vi "test2.vi"() -> ()   [LabVIEW 2019]
uses:
  <vilib>/measure/NI_MABase.lvlib
panel:
  out "Button 2":dbl
  out "Button 1":dbl
  out "Y":dbl
  out "X":dbl
  in  "Frequeny":dbl(slide) scale=0.0..10.0
  in  "Amplitude":dbl(slide) scale=0.0..10.0
  in  "Power":bool
  out "Signal":dynamicdata(graph)
  in  "Sine":bool
  # "Remote gesture control enabled Control Panel"
  # "Square"
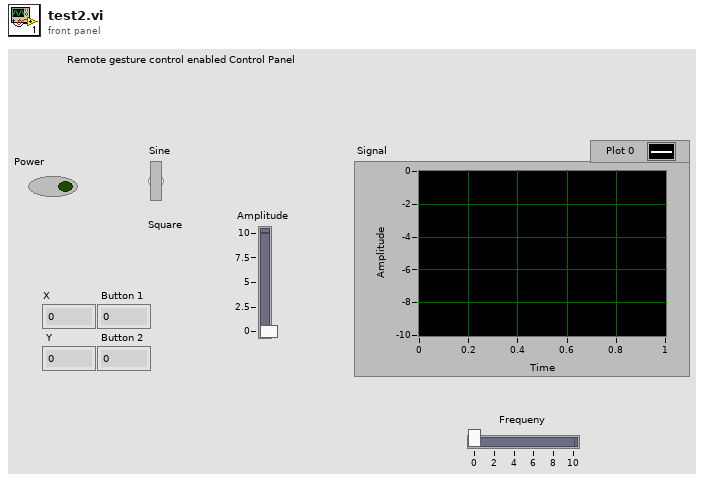
[diagram p1: front panel]
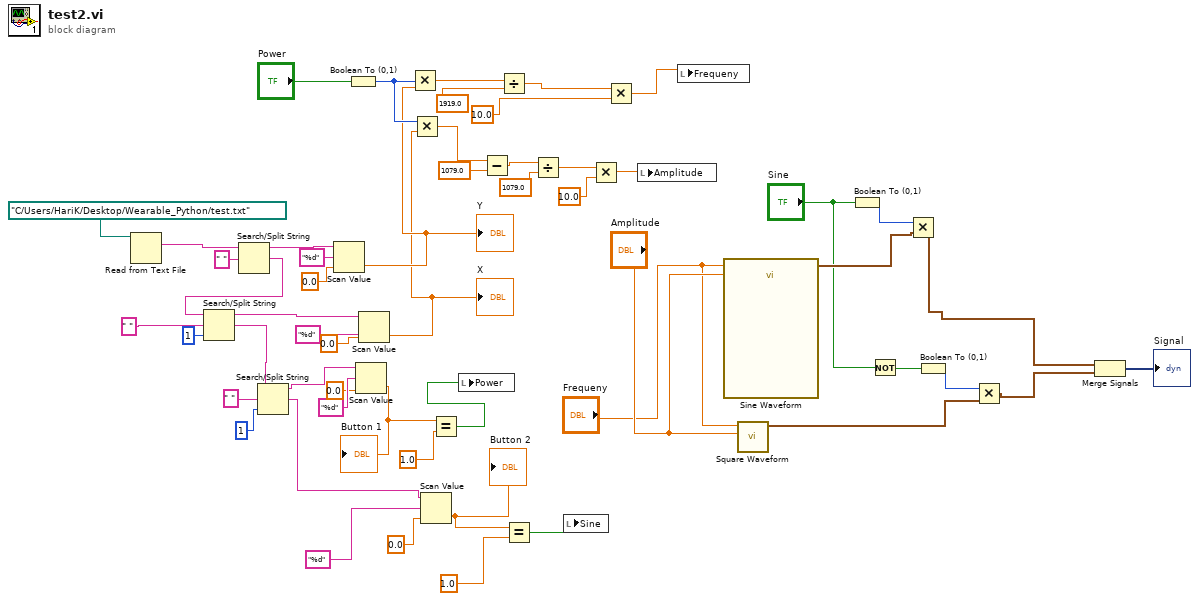
[diagram p0: block diagram]
diagram:
  n1 = Read from Text File(file (use dialog)=path "C:/Users/HariK/Desktop/Wearable_Python/test.txt") -> (text=w41:string)  [unwired: 3 in, 3 out]
  n2 = Search/Split String(string=w41, search string/char (-)=" ") -> (substring before match=w31:string, match + rest of string=w15:string)  [unwired: 1 in, 1 out]
  n3 = Search/Split String(string=w15, search string/char (-)=" ", offset (0)=1) -> (substring before match=w29:string, match + rest of string=w39:string)  [unwired: 1 out]
  n4 = Search/Split String(string=w39, search string/char (-)=" ", offset (0)=1) -> (substring before match=w36:string, match + rest of string=w17:string)  [unwired: 1 out]
  n5 = Scan Value(string=w31, format string="%d", default (0 dbl)=0.0) -> (value=w27:dbl)  [unwired: 1 out]
  "Y" <- w27
  n6 = Boolean To (0,1)(Boolean="Power") -> (0, 1=w37:i16)
  n7 = Scan Value(string=w36, format string="%d", default (0 dbl)=0.0) -> (value=w21:dbl)  [unwired: 1 out]
  "Button 1" <- w21
  n8 = Scan Value(string=w29, format string="%d", default (0 dbl)=0.0) -> (value=w26:dbl)  [unwired: 1 out]
  "X" <- w26
  n9 = Multiply(x=w37, y=w27) -> (x*y=w2:dbl)
  n10 = Multiply(x=w37, y=w26) -> (x*y=w11:dbl)
  n11 = Scan Value(string=w17, format string="%d", default (0 dbl)=0.0) -> (value=w25:dbl)  [unwired: 1 out]
  "Button 2" <- w25
  n12 = Equal?(x=w21, y=1.0) -> (x = y?=w20:bool)
  n13 = local write "Power"(w20) -> ()
  n14 = Subtract(x=w11, y=1079.0) -> (x-y=w10:dbl)
  n15 = Divide(x=w2, y=1919.0) -> (x/y=w4:dbl)
  n16 = Equal?(x=w25, y=1.0) -> (x = y?=w23:bool)
  n17 = Divide(x=w10, y=1079.0) -> (x/y=w8:dbl)
  n18 = local write "Sine"(w23) -> ()
  n19 = Multiply(x=w8, y=10.0) -> (x*y=w6:dbl)
  n20 = Multiply(x=w4, y=10.0) -> (x*y=w1:dbl)
  n21 = local write "Amplitude"(w6) -> ()
  n22 = local write "Frequeny"(w1) -> ()
  n23 = call <vilib>:"Sine Waveform.vi"("amplitude"="Amplitude", "frequency"="Frequeny") -> ("signal out"=w49:waveform(dbl))  [unwired: 8 in, 1 out]
  n24 = call <vilib>:"Square Waveform.vi"("amplitude"="Amplitude", "frequency"="Frequeny") -> ("signal out"=w45:waveform(dbl))  [unwired: 8 in, 1 out]
  n25 = Boolean To (0,1)(Boolean="Sine") -> (0, 1=w50:i16)
  n26 = Not(x="Sine") -> (.not. x?=w46:bool)
  n27 = Multiply(x=w50, y=w49) -> (x*y=w43:waveform(dbl))
  n28 = Boolean To (0,1)(Boolean=w46) -> (0, 1=w47:i16)
  n29 = Multiply(x=w47, y=w45) -> (x*y=w44:waveform(dbl))
  n30 = Merge Signals(w43, w44) -> (→"Signal":dynamicdata)
